vi "sample-profiled-pid-turn-to-angle-execute.vi"() -> ()   [LabVIEW 2019]
uses:
  <vilib>/Rock Robotics/WPI/ThirdParty/JAS_Junk/TrajLib/LinearFilter_ResetToValue.vi
  <vilib>/Rock Robotics/WPI/ThirdParty/JAS_Junk/TrajLib/LinearFilter_Calculate.vi
  <vilib>/Rock Robotics/WPI/ThirdParty/JAS_Junk/TrajLib/ProfiledPIDController_SetPID.vi
  <vilib>/Rock Robotics/WPI/ThirdParty/JAS_Junk/TrajLib/ProfiledPIDController_SetIntegratorRange.vi
  <vilib>/Rock Robotics/WPI/ThirdParty/JAS_Junk/TrajLib/ProfiledPIDController_SetTolerance_PosVel.vi
  <vilib>/Rock Robotics/WPI/ThirdParty/JAS_Junk/TrajLib/ProfiledPIDController_DisableContInput.vi
  <vilib>/Rock Robotics/WPI/ThirdParty/JAS_Junk/TrajLib/ProfiledPIDController_EnableContInput.vi
  <vilib>/Rock Robotics/WPI/ThirdParty/JAS_Junk/TrajLib/ProfiledPIDController_Reset_PosOnly.vi
  <vilib>/Rock Robotics/WPI/ThirdParty/JAS_Junk/TrajLib/ProfiledPIDController_NewPeriod.vi
  <vilib>/Rock Robotics/WPI/ThirdParty/JAS_Junk/TrajLib/ProfiledPIDController_Calculate_Meas_Goal.vi
  <vilib>/Rock Robotics/WPI/ThirdParty/JAS_Junk/TrajLib/ProfiledPIDController_AtGoal.vi
  <vilib>/Rock Robotics/WPI/ThirdParty/JAS_Junk/TrajLib/ProfiledPIDController_AtSetpoint.vi
  <vilib>/Rock Robotics/WPI/ThirdParty/JAS_Junk/TrajLib/ProfiledPIDController_SetConstraints.vi
  <vilib>/Rock Robotics/WPI/ThirdParty/JAS_Junk/TrajLib/PIDController_GetVelocityError.vi
  <vilib>/Rock Robotics/WPI/ThirdParty/JAS_Junk/TrajLib/PIDController_GetPositionError.vi
  <vilib>/Rock Robotics/WPI/ThirdParty/JAS_Junk/TrajLib/PIDController_SetPID.vi
  <vilib>/Rock Robotics/WPI/ThirdParty/JAS_Junk/TrajLib/PIDController_SetIntegratorRange.vi
  <vilib>/Rock Robotics/WPI/ThirdParty/JAS_Junk/TrajLib/PIDController_SetTolerancePandV.vi
  <vilib>/Rock Robotics/WPI/ThirdParty/JAS_Junk/TrajLib/PIDController_DisableContinousInput.vi
  <vilib>/Rock Robotics/WPI/ThirdParty/JAS_Junk/TrajLib/PIDController_EnableContinousInput.vi
  <vilib>/Rock Robotics/WPI/ThirdParty/JAS_Junk/TrajLib/TrapProfState_New.vi
  <vilib>/Rock Robotics/WPI/ThirdParty/JAS_Junk/TrajLib/ProfiledPIDController_Reset.vi
  <vilib>/Rock Robotics/WPI/ThirdParty/JAS_Junk/TrajLib/PIDController_NewPeriod.vi
  <vilib>/Rock Robotics/SystemInterfaces/NetworkCommunication/NetComm_UsageReport_report.vi
  <vilib>/Rock Robotics/WPI/ThirdParty/JAS_Junk/TrajLib/ProfiledPIDController_SetGoal_PosOnly.vi
  <vilib>/Rock Robotics/WPI/ThirdParty/JAS_Junk/TrajLib/ProfiledPIDController_Calculate_Meas.vi
  <vilib>/Rock Robotics/WPI/ThirdParty/JAS_Junk/TrajLib/TrapProfState_Equals.vi
  <vilib>/Rock Robotics/WPI/ThirdParty/JAS_Junk/TrajLib/PIDController_AtSetpoint.vi
  <vilib>/Rock Robotics/WPI/ThirdParty/JAS_Junk/TrajLib/PIDController_Reset.vi
  <vilib>/Rock Robotics/WPI/ThirdParty/JAS_Junk/TrajLib/ProfiledPIDController_SetGoal.vi
  <vilib>/Rock Robotics/WPI/ThirdParty/JAS_Junk/TrajLib/PIDController_Calculate_SP_PV.vi
  <vilib>/Rock Robotics/WPI/ThirdParty/JAS_Junk/TrajLib/TrapProfile_New.vi
  <vilib>/Rock Robotics/WPI/ThirdParty/JAS_Junk/TrajLib/ProfiledPIDController_GetPeriod.vi
  <vilib>/Rock Robotics/WPI/ThirdParty/JAS_Junk/TrajLib/TrapProfile_Calculate.vi
  <vilib>/Rock Robotics/WPI/ThirdParty/JAS_Junk/TrajLib/ControllerUtil_GetModulusError.vi
  <vilib>/Rock Robotics/WPI/ThirdParty/JAS_Junk/TrajLib/PIDController_SetSetpoint.vi
  <vilib>/Rock Robotics/WPI/ThirdParty/JAS_Junk/TrajLib/PIDController_Calculate_PV.vi
  <vilib>/Rock Robotics/WPI/ThirdParty/JAS_Junk/TrajLib/TrapProfile_ShouldFlipAcceleration.vi
  <vilib>/Rock Robotics/WPI/ThirdParty/JAS_Junk/TrajLib/TrapProfile_Direct.vi
  <vilib>/Rock Robotics/WPI/ThirdParty/JAS_Junk/TrajLib/PIDController_GetPeriod.vi
  <vilib>/Rock Robotics/WPI/ThirdParty/JAS_Junk/TrajLib/LinearFilter_MovingAverage.vi
  <vilib>/Rock Robotics/WPI/ThirdParty/JAS_Junk/TrajLib/LinearFilter_LowPassBW1.vi
  <vilib>/Rock Robotics/WPI/ThirdParty/JAS_Junk/TrajLib/LinearFilter_LowPassBW2.vi
  <vilib>/Rock Robotics/WPI/ThirdParty/JAS_Junk/TrajLib/LinearFilter_HighPassBW1.vi
  <vilib>/Rock Robotics/WPI/ThirdParty/JAS_Junk/TrajLib/LinearFilter_HighPassBW2.vi
  <vilib>/Rock Robotics/WPI/ThirdParty/JAS_Junk/TrajLib/Util_LibraryGlobals.vi
  <vilib>/Rock Robotics/WPI/ThirdParty/JAS_Junk/TrajLib/Trajectory_Library.lvlib
  <vilib>/ptbypt/NI_PtbyPt.lvlib
panel:
  in  "Tab Control":enum32{"Operation", "Tuning"}(tab)
  out "Targets along the way":T1(graph)
  in  "SP - Desired Angle\n (Deg)":dbl(slide) scale=-10.0..350.0
  out "PV - Current Angle\n (Deg)":dbl(slide) scale=-10.0..350.0
  out "Goal Chart":T2(graph)
  out "Motor Output":dbl format="%13.3f"
  out "AtSetpoint":bool
  out "AtGoal":bool
  out "PositionError  (Deg)":dbl format="%13.2f"
  out "VelocityError  (Deg/Sec)":dbl format="%13.2f"
  out "Velocity  (Deg/Sec)":dbl format="%13.2f"
  in  "Kp":dbl=0.08 format="%#_13g"
  in  "Ki":dbl=0.15 format="%#_13g"
  in  "Kd":dbl format="%#_13g"
  in  "Minimum Integral":dbl=-0.3 format="%#_13g"
  in  "Maximum Integral":dbl=0.3 format="%#_13g"
  in  "Max Speed   (Deg/Sec)":dbl=30.0 format="%#_13g"
  in  "Max Accel  (Deg/Sec^2)":dbl=5.0 format="%#_13g"
  in  "PositionTolerance\n(Deg)":dbl=1.0 format="%#_13g"
  in  "VelocityTolerance\n(Deg/Sec)":dbl=0.05 format="%#_13g"
  # "PID Tuning Parameters"
  # "Desired Profile Performance"
  # "Desired On Target Tolerance"
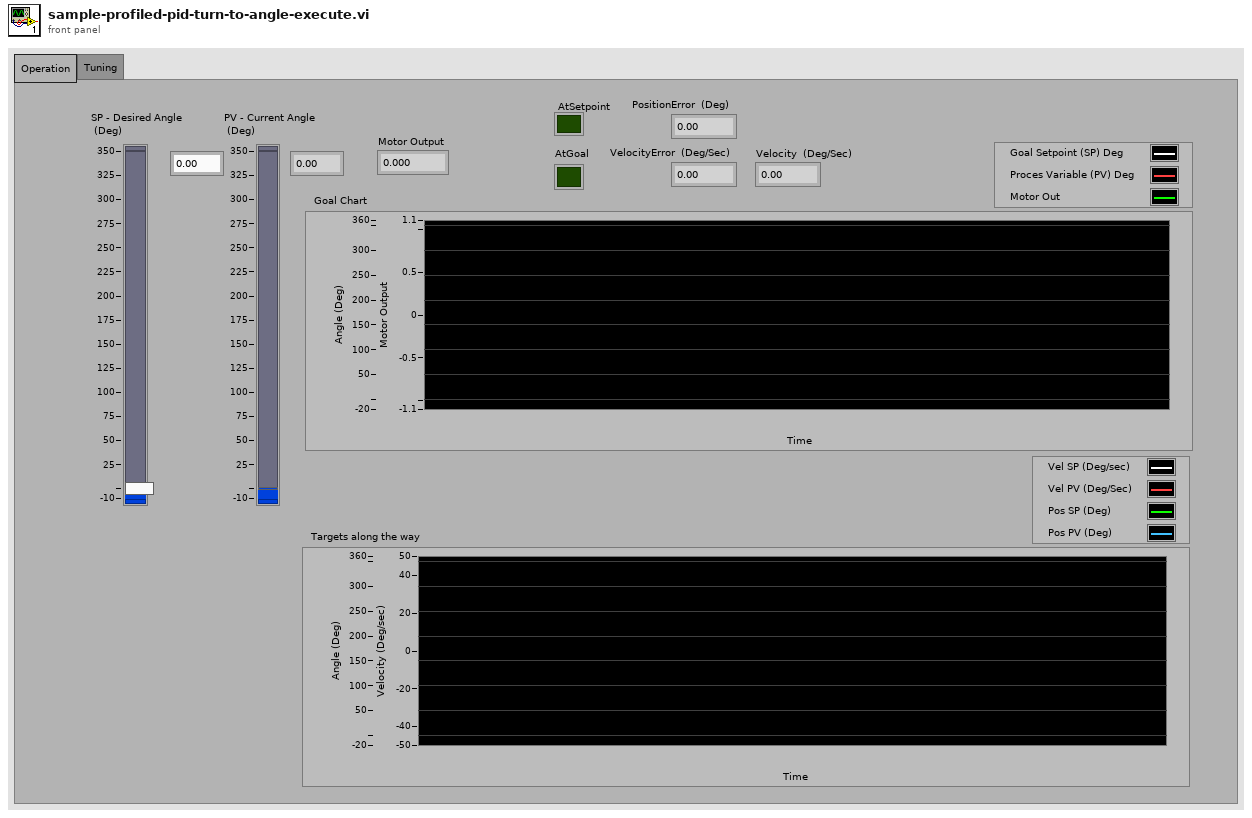
[diagram p1: front panel]
types:
  T1 = cluster{"SP - Desired Heading\n (Deg)":dbl, "PV - Current Heading\n (Deg)":dbl, "upper limit":dbl, dbl}
  T2 = cluster{"SP - Desired Position\n (Inch)":dbl, "upper limit":dbl, "upper limit":dbl}
  T3 = enum16{"Moving Average", "Low Pass 1st Order Butterworth", "Low Pass 2nd Order Butterworth", "High Pass 1st Order Butterworth", "High Pass 2nd Order Butterworth"}
  T4 = typedef "Trajectory_Library.lvlib/PID_ERROR_TOLERANCE.ctl" = cluster{"PositionTolerance":dbl, "VelocityTolerance":dbl}
  T5 = typedef "Trajectory_Library.lvlib/PID_TUNING.ctl" = cluster{"Kp":dbl, "Ki":dbl, "Kd":dbl, "MaximumIntegral":dbl, "MinimumIntegral":dbl}
  T6 = typedef "Trajectory_Library.lvlib/PID_INPUT_LIMITS.ctl" = cluster{"MaxInput":dbl, "MinInput":dbl, "Continuous":bool}
  T7 = typedef "Trajectory_Library.lvlib/TRAPEZOID_PROFILE_CONSTRAINT.ctl" = cluster{"MaxVelocity":dbl, "MaxAcceleration":dbl}
  T8 = typedef "Trajectory_Library.lvlib/PROFILED_PID_CONTROLLER.ctl" = cluster{"Controller":T9, "Goal":T10, "Setpoint":T10, "Constraint":T7}
  T9 = typedef "Trajectory_Library.lvlib/PID_CONTROLLER.ctl" = cluster{"Kp":dbl, "Ki":dbl, "Kd":dbl, "Period":dbl, "Max_Integral":dbl, "Min_Integral":dbl, "Max_Input":dbl, "Min_Input":dbl, "Continuous":bool, "PositionError":dbl, "VelocityError":dbl, "PrevError":dbl, "TotalError":dbl, "PositionTolerance":dbl, "VelocityTolerance":dbl, "SetPoint":dbl, "Kf":dbl, "Prev_Deriv":dbl, "Prev_Deriv 2":dbl, "DerivativeFilter":bool, "Min_Output":dbl, "Max_Output":dbl, "Prev_F_P":dbl, "Prev_F_P_2":dbl, "AntiWindupActive":bool, "Measurement":dbl}
  T10 = typedef "Trajectory_Library.lvlib/TRAPEZOID_PROFILE_STATE.ctl" = cluster{"Position":dbl, "Velocity":dbl}
  T11 = cluster{"SP - Desired Angle\n (Deg)":dbl, "modulus":dbl, "upper limit":dbl}
  T12 = cluster{"Velocity":dbl, dbl, "Position":dbl, "modulus":dbl}
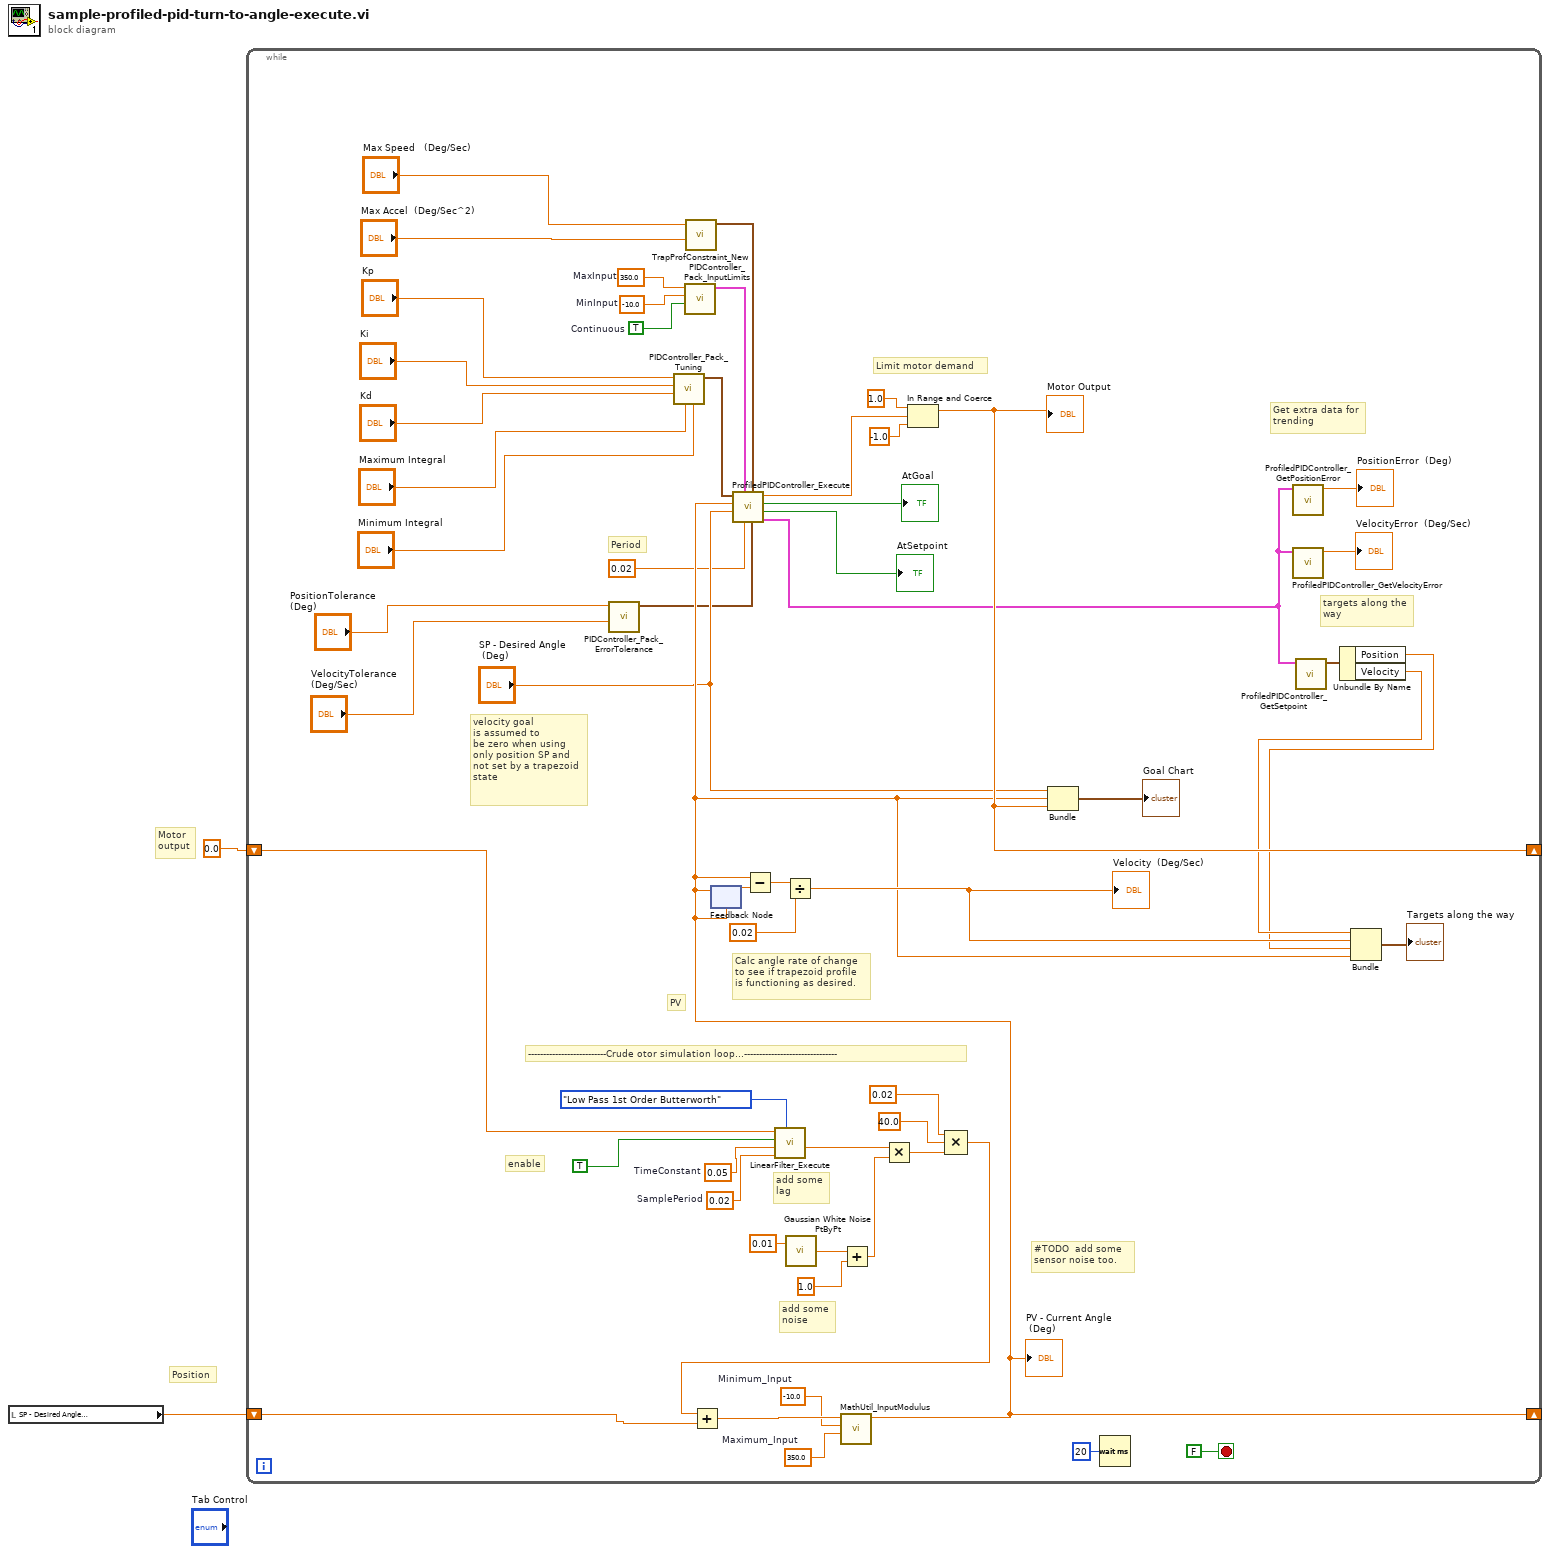
[diagram p0: block diagram]
diagram:
  # "Position"
  # "Motor\noutput"
  n1 = local read "SP - Desired Angle\n (Deg)"() -> (w1:dbl)
  n2 = while {
    shift-right: [w19] -> _
    shift-left: w1 -> [w37]
    shift-right: [w36] -> _
    shift-left: 0.0 ("upper limit") -> [w35]
    stop <- FALSE stop-if-true
    w24 = 350.0  # MaxInput
    w23 = -10.0  # MinInput
    w22 = TRUE  # Continuous
    w26 = -10.0  # Minimum_Input
    w27 = 350.0  # Maximum_Input
    w39 = 0.02  # SamplePeriod
    w38 = 0.05  # TimeConstant
    # "Get extra data for\ntrending"
    # "Period"
    # "Limit motor demand"
    # "targets along the\nway"
    # "enable"
    # "PV"
    # "#TODO  add some\nsensor noise too."
    # "add some\nnoise"
    # "add some\nlag"
    # "--------------------------Crude otor simulation loop...-------------------------------"
    # "Calc angle rate of change\nto see if trapezoid profile\nis functioning as desired."
    # "velocity goal\nis assumed to \nbe zero when using\nonly position SP and\nnot set by a trapezoid\nstate"
    n3 = call <vilib>:"PIDController_Pack_ErrorTolerance.vi"("VelocityTolerance"="VelocityTolerance\n(Deg/Sec)", "PositionTolerance"="PositionTolerance\n(Deg)") -> ("PID Error Tolerance"=w3:T4)  [unwired: 9 in]
    n4 = call <vilib>:"PIDController_Pack_Tuning.vi"("MinimumIntegral"="Minimum Integral", "MaximumIntegral"="Maximum Integral", "Kd"="Kd", "Ki"="Ki", "Kp"="Kp") -> ("PID Tuning"=w21:T5)  [unwired: 6 in]
    n5 = call <vilib>:"PIDController_Pack_InputLimits.vi"("Continuous"=w22, "MinInput"=w23, "MaxInput"=w24) -> ("PID Input Limits"=w20:T6)  [unwired: 8 in]
    n6 = call <vilib>:"TrapProfConstraint_New.vi"("Max Accel"="Max Accel  (Deg/Sec^2)", "Max Speed (M/S)"="Max Speed   (Deg/Sec)") -> ("TRAPEZOID_PROFILE_CONSTRAINT"=w25:T7)  [unwired: 9 in]
    n7 = call <vilib>:"LinearFilter_Execute.vi"("Filter Type"=T3."Low Pass 1st Order Butterworth", "SamplePeriod"=w39, "TimeConstant"=w38, "Enable"=TRUE, "Input"=w35) -> ("Output"=w46:dbl)  [unwired: 5 in, 1 out]
    n8 = call <vilib>:"Gaussian White Noise PtByPt.vi"("standard deviation"=0.01) -> ("Gaussian white noise"=w45:dbl)  [unwired: 2 in]
    n9 = Add(x=w45, y=1.0) -> (x+y=w47:dbl)
    n10 = Multiply(x=w46, y=w47) -> (x*y=w48:dbl)
    n11 = Compound Arithmetic op=MULTIPLY(0.02 ("value"), 40.0 ("value"), w48) -> (w49:dbl)
    n12 = Add(x=w49, y=w37) -> (x+y=w28:dbl)
    n13 = call <vilib>:"MathUtil_InputModulus.vi"("Maximum_Input"=w27, "Minimum_Input"=w26, "Input"=w28) -> ("modulus"=w19:dbl)  [unwired: 8 in]
    "PV - Current Angle\n (Deg)" <- w19
    n14 = feedback-in #1(w19) -> ()
    n15 = feedback #1(w19) -> (w55:dbl)
    n16 = call <vilib>:"ProfiledPIDController_Execute.vi"("PID Error Tolerance"=w3, "Constraints"=w25, "Period"=0.02, "PID Input Limits"=w20, "SP-SetPoint Goal"="SP - Desired Angle\n (Deg)", "PV-Measurement"=w19, "PID Tuning"=w21) -> ("out PID_CONTROLLER"=w14:T8, "AtSetpoint"=→"AtSetpoint":bool, "AtGoal"=→"AtGoal":bool, "CO-ControlOutput"=w17:dbl)  [unwired: 1 in]
    n17 = Subtract(x=w19, y=w55) -> (x-y=w54:dbl)
    n18 = Divide(x=w54, y=0.02) -> (x/y=w30:dbl)
    "Velocity  (Deg/Sec)" <- w30
    n19 = In Range and Coerce(upper limit=1.0, x=w17, lower limit=-1.0) -> (coerced(x)=w36:dbl)  [unwired: 1 out]
    "Motor Output" <- w36
    n20 = Bundle("SP - Desired Angle\n (Deg)"="SP - Desired Angle\n (Deg)", "modulus"=w19, "upper limit"=w36) -> (→"Goal Chart":T11)  [unwired: 1 in]
    n21 = Wait (ms)(milliseconds to wait=u32 20) -> ()  [unwired: 1 out]
    n22 = call <vilib>:"ProfiledPIDController_GetPositionError.vi"("in PROFILED_PID_CONTROLLER"=w14) -> ("PositionError"=→"PositionError  (Deg)":dbl)  [unwired: 10 in]
    n23 = call <vilib>:"ProfiledPIDController_GetVelocityError.vi"("in PROFILED_PID_CONTROLLER"=w14) -> ("VelocityError"=→"VelocityError  (Deg/Sec)":dbl)  [unwired: 10 in]
    n24 = call <vilib>:"ProfiledPIDController_GetSetpoint.vi"("in PROFILED_PID_CONTROLLER"=w14) -> ("Setpoint"=w32:T10)  [unwired: 10 in]
    n25 = Unbundle By Name(w32) -> ("Position"=w29:dbl, "Velocity"=w31:dbl)
    n26 = Bundle("Velocity"=w31, w30, "Position"=w29, "modulus"=w19) -> (→"Targets along the way":T12)  [unwired: 1 in]
  }
